vi "Rising Edge Detect.vi"(11 "Input":bool) -> (3 "Rising Edge":bool)   [LabVIEW 2012]
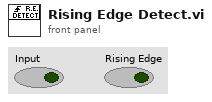
[diagram p1: front panel]
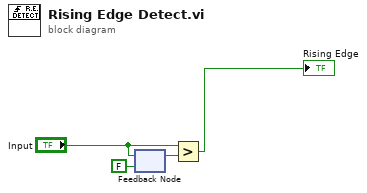
[diagram p0: block diagram]
diagram:
  n1 = feedback #1(FALSE) -> (w3:bool)
  n2 = feedback-in #1("Input") -> ()
  n3 = Greater?(x="Input", y=w3) -> (0:→"Rising Edge":bool)
